vi "DT_Cal Triangle Area.vi"(9 "p 3":cluster{"x":dbl, "y":dbl, "index":i32}, 10 "p 2":cluster{"x":dbl, "y":dbl, "index":i32}, 11 "p 1":cluster{"x":dbl, "y":dbl, "index":i32}) -> (3 "area":dbl)   [LabVIEW 2020, in "NI_AAL_Geometry.lvlib"]
uses:
  <vilib>/Analysis/NI_AAL_Geometry.lvlib
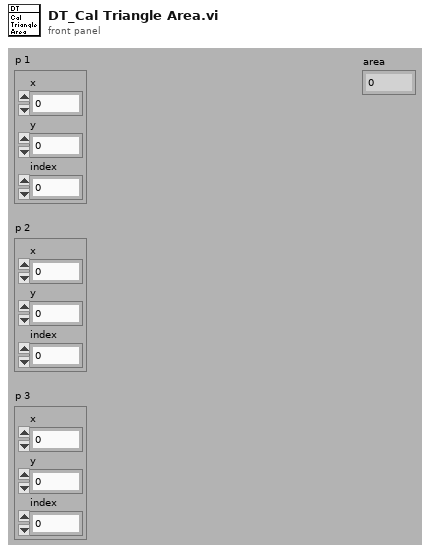
[diagram p1: front panel]
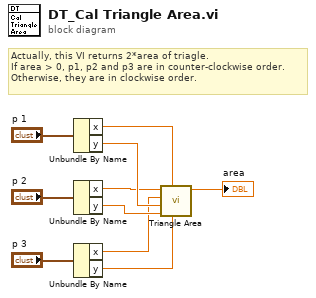
[diagram p0: block diagram]
diagram:
  # "Actually, this VI returns 2*area of triagle.\nIf area > 0, p1, p2 and p3 are in counter-clockwise order.\nOtherwise, they are in clockwise order."
  n1 = Unbundle By Name("p 1") -> ("x"=w9:dbl, "y"=w8:dbl)
  n2 = Unbundle By Name("p 2") -> ("x"=w6:dbl, "y"=w5:dbl)
  n3 = Unbundle By Name("p 3") -> ("x"=w3:dbl, "y"=w2:dbl)
  n4 = call <vilib>:"Triangle Area.vi"("y 3"=w2, "x 1"=w9, "y 2"=w5, "y 1"=w8, "x 3"=w3, "x 2"=w6) -> ("area"=→"area":dbl)  [unwired: 5 in]
